vi "GetTandH.vi"(8 "error in (no error)":errorcluster, 11 "Temperhum.Thorlabs in":refnum<class "Temperhum.Thorlabs.lvclass">) -> (0 "error out":errorcluster, 1 "Humidity (%RH)":dbl, 2 "Temperature (K)":dbl, 3 "Temperhum.Thorlabs out":refnum<class "Temperhum.Thorlabs.lvclass">)   [LabVIEW 2019, in "Temperhum.Thorlabs.lvclass"]
uses:
  Temperhum.Thorlabs.lvclass
  Temperhum.Thorlabs.lvclass/Temperhum.Thorlabs.ctl
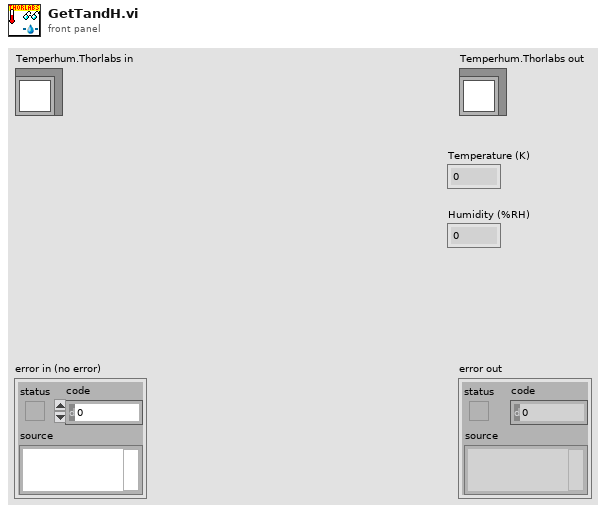
[diagram p1: front panel]
types:
  T1 = typedef "Temperhum.Thorlabs.lvclass/Thorlabs Type --enum.ctl" = enum16{"A", "B"}
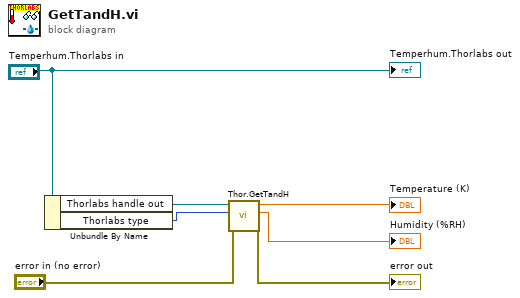
[diagram p0: block diagram]
diagram:
  n1 = Unbundle By Name("Temperhum.Thorlabs in") -> ("Thorlabs handle out"=w3:refnum<visa-resource-name>, "Thorlabs type"=w1:T1)
  n2 = call "Thor.GetTandH.vi"("error in (no error)"="error in (no error)", "Thorlabs type"=w1, "Thorlabs handle out"=w3) -> ("error out"=→"error out":errorcluster, "Humidity"=→"Humidity (%RH)":dbl, "Temperature"=→"Temperature (K)":dbl)  [unwired: 6 in]
  "Temperhum.Thorlabs out" <- "Temperhum.Thorlabs in"
